vi "_Standardize Carriage Returns.vi"(11 "States":string) -> (3 "trimed text":string)   [LabVIEW 2017, in "csmdoc.lvlib"]
uses:
  csmdoc.lvlib
  _Shared/CSM Shared.lvlib
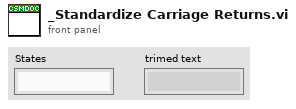
[diagram p1: front panel]
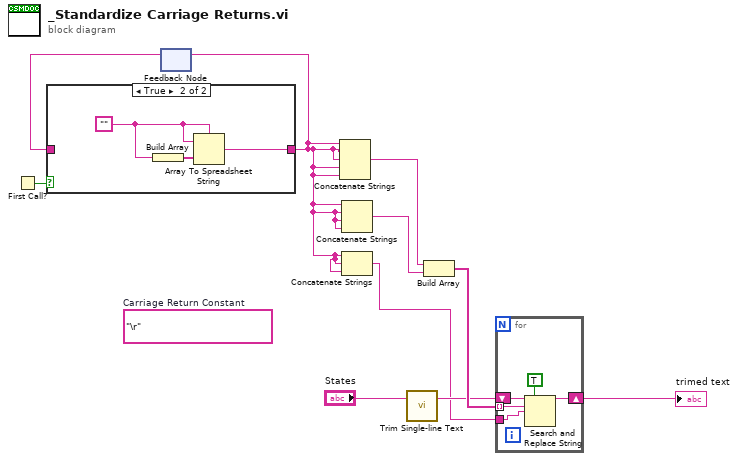
[diagram p0: block diagram]
diagram:
  (unwired) "\r"  # Carriage Return Constant
  n1 = First Call?() -> (First Call?: T/F=w6:bool)
  n2 = feedback #1() -> (w7:string)  [unwired: 1 in]
  n3 = case shown="True" w6 {
    tunnel: [w11 w12] -> w10
    tunnel: w7 -> [w11 _]
    frame False {
    }
    frame True {
      w13 = "" ("Empty String\n(hidden on FP)")
      n4 = Build Array(w13) -> (w14:string[])
      n5 = Array To Spreadsheet String(delimiter (Tab)=w13, array=w14, 3:w13) -> (spreadsheet string=w12:string)
    }
  }
  n6 = feedback-in #1(w10) -> ()
  n7 = Concatenate Strings(w10, w10, w10, w10, w10) -> (w8:string)
  n8 = Concatenate Strings(w10, w10, w10, w10) -> (w9:string)
  n9 = Concatenate Strings(w10, w10, w10) -> (w1:string)
  n10 = call "Trim Single-line Text.vi"("single-line text"="States") -> ("trimed text"=w4:string)  [unwired: 2 in]
  n11 = Build Array(w8, w9) -> (w5:string[])
  n12 = for {
    shift-right: [w19] -> w3
    shift-left: w4 -> [w18]
    tunnel: w5 -> [w16] mode=indexing
    tunnel: w1 -> [w15]
    n13 = Search and Replace String(replace all?=TRUE ("replace all? (F)"), input string=w18, search string=w16, replace string=w15) -> (result string=w19:string)  [unwired: 4 in, 3 out]
  }
  "trimed text" <- w3
